vi "pkyk_text_img.vi"(4 "Fill Color":u32, 5 "[user-specified font]":T2, 6 "Text Color":u32, 7 "Column":i16=10, 9 "Text":string, 10 "Orgin In":T1, 11 "new picture in":picture) -> (2 "Orgin Out":T1, 3 "new picture out":picture)   [LabVIEW 2020]
uses:
  <vilib>/picture/picture.llb/Draw True-Color Pixmap.vi
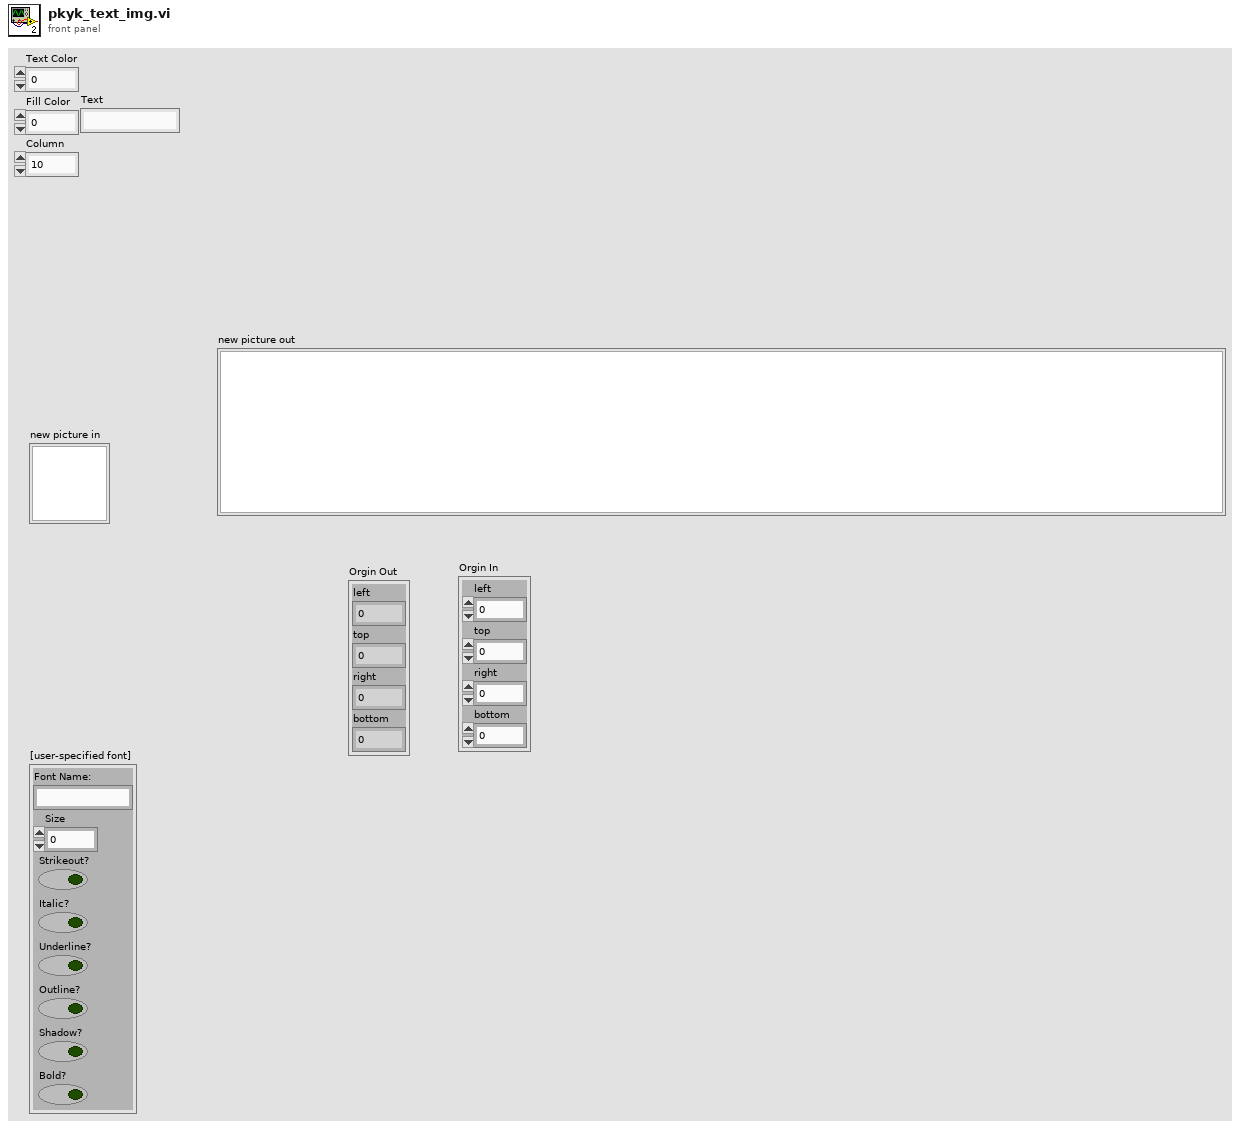
[diagram p1: front panel]
types:
  T1 = cluster{"left":i16, "top":i16, "right":i16, "bottom":i16}
  T2 = cluster{"Font Name:":string, "Size":i16, "Strikeout?":bool, "Italic?":bool, "Underline?":bool, "Outline?":bool, "Shadow?":bool, "Bold?":bool}
  T3 = enum16{"User-specified Font", "Application Font", "System Font", "Dialog Font"}
  T4 = typedef "imagedata.ctl" = cluster{"image type":i32, "image depth":i32, "image":u8[], "mask":u8[], "colors":u32[], "Rectangle":cluster{"left":i16, "top":i16, "right":i16, "bottom":i16}}
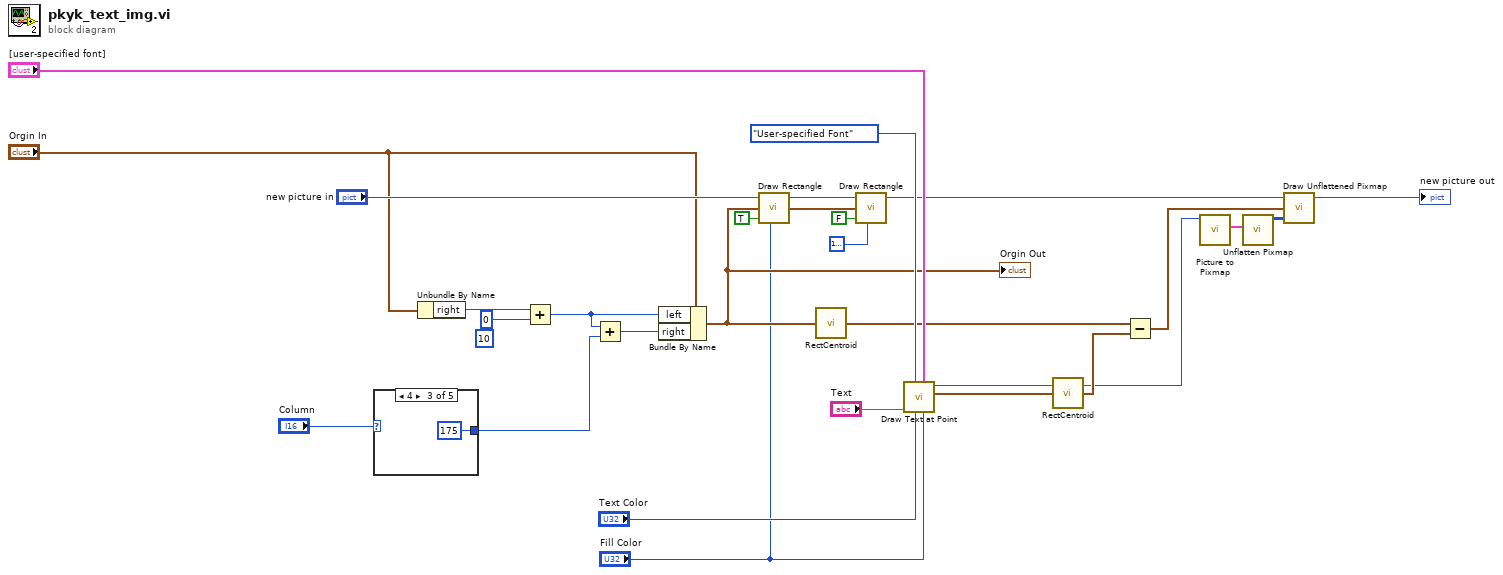
[diagram p0: block diagram]
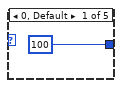
[diagram p2: hidden frame]
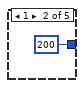
[diagram p3: hidden frame]
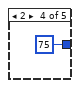
[diagram p4: hidden frame]
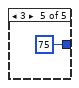
[diagram p5: hidden frame]
diagram:
  (unwired) i16 10 ("x")
  n1 = case shown="4" "Column" {
    tunnel: [i16 100 ("right") i16 200 ("right") i16 175 ("right") i16 75 ("right") i16 75 ("right")] -> w24
    frame 0, Default {
    }
    frame 1 {
    }
    frame 4 {
    }
    frame 2 {
    }
    frame 3 {
    }
  }
  n2 = Unbundle By Name("Orgin In") -> ("right"=w22:i16)
  n3 = Add(x=w22, y=i16 0 ("x")) -> (x+y=w1:i16)
  n4 = Add(x=w1, y=w24) -> (x+y=w25:i16)
  n5 = Bundle By Name(cluster="Orgin In", "left"=w1, "right"=w25) -> (w6:T1)
  "Orgin Out" <- w6
  n6 = call <vilib>:"Draw Rectangle.vi"("picture"="new picture in", "rect"=w6, "fill?(F)"=TRUE, "color(black)"="Fill Color") -> ("new picture"=w19:picture)  [unwired: 5 in]
  n7 = call <vilib>:"RectCentroid.vi"("rect"=w6) -> ("point"=w15:cluster{"x":i16, "y":i16})
  n8 = call <vilib>:"Draw Rectangle.vi"("picture"=w19, "rect"=w6, "fill?(F)"=FALSE, "color(black)"=u32 16777222) -> ("new picture"=w9:picture)  [unwired: 5 in]
  n9 = call <vilib>:"Draw Text at Point.vi"("BG color(transparent)"="Fill Color", "[user-specified font]"="[user-specified font]", "text color(black)"="Text Color", "desired font(Application)"=T3."User-specified Font", "text"="Text") -> ("text rect"=w14:T1, "new picture"=w12:picture)  [unwired: 5 in]
  n10 = call <vilib>:"RectCentroid.vi"("rect"=w14) -> ("point"=w13:cluster{"x":i16, "y":i16})
  n11 = Subtract(x=w15, y=w13) -> (x-y=w8:cluster{"x":i16, "y":i16})
  n12 = call <vilib>:"Picture to Pixmap.vi"("picture"=w12) -> ("image data"=w11:T4)  [unwired: 9 in, 1 out]
  n13 = call <vilib>:"Unflatten Pixmap.vi"("image data"=w11) -> ("24-bit pixmap"=w10:u32[][])  [unwired: 4 in, 6 out]
  n14 = call-poly <vilib>:"Draw Unflattened Pixmap.vi"("picture"=w9, "top left point(0, 0)"=w8, "data (RGB format)"=w10) -> ("new picture"=→"new picture out":picture)  [unwired: 6 in]
